vi "IMAQdx Serial Write.vi"(7 "Timeout (ms)":u32=1000, 8 "error in":errorcluster, 10 "Data":string, 11 "Session In":T1) -> (0 "error out":errorcluster, 3 "Session Out":T1)   [LabVIEW 2020, in "NI_Vision_Acquisition_Software.lvlib"]
doc: "Writes data to the serial port."
uses:
  NI_Vision_Acquisition_Software.lvlib
  IMAQdx.ctl
  niimaqdx.dll
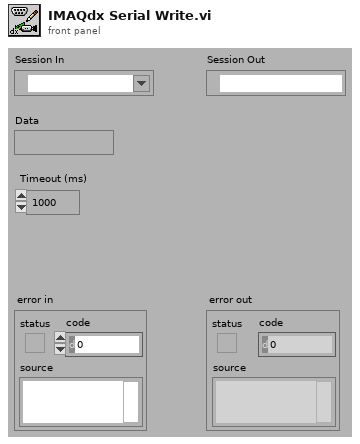
[diagram p1: front panel]
types:
  T1 = typedef "IMAQdx.ctl" = refnum<k21>
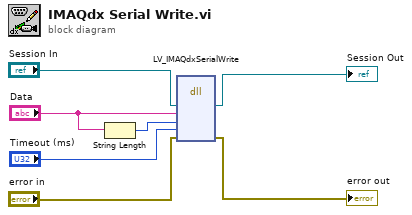
[diagram p0: block diagram]
diagram:
  n1 = String Length(string="Data") -> (length=w6:i32)
  n2 = dll-call lib="niimaqdx.dll" fn="LV_IMAQdxSerialWrite"("refnum"="Session In", "StringToWrite"="Data", "StringSize"=w6, "Timeout"="Timeout (ms)", "error"="error in") -> ("refnum"=→"Session Out":T1, "error"=→"error out":errorcluster)  [unwired: 6 in, 3 out]
